vi "Global_Variables.vi"() -> ()   [LabVIEW 2021]
panel:
  in  "Slow - Servo Y":dbl
  in  "Slow - ServoX":dbl
  in  "Automatic":bool
  in  "session out":refnum<k35>
  out "appended path":path
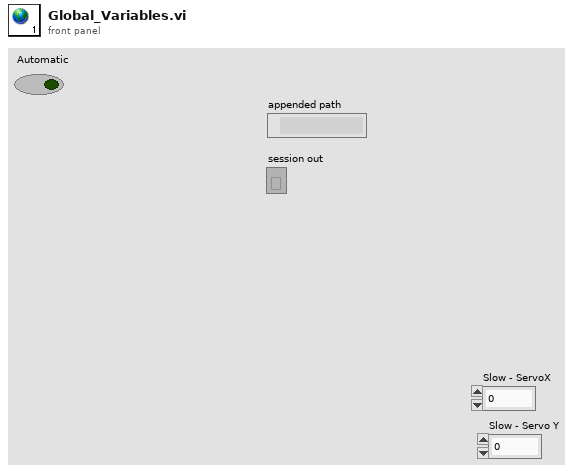
[diagram p1: front panel]
diagram:
